vi "Wait for Record Event.vi"(6 "Cancel":bool, 8 "error in":errorcluster, 9 "Timeout in ms (0: infinite)":u32, 10 "Event":u16(ring)=32 items=["Record Start"=32, "Record End"=64, "Start Trigger"=128], 11 "VISA resource name":refnum<visa-resource-name>) -> (0 "error out":errorcluster, 3 "VISA resource name out":refnum<visa-resource-name>)   [LabVIEW 2017, in "Sefram DAS220.lvlib"]
doc: "Wait for record event : start, end or start trigger."
uses:
  <instrlib>/Sefram DAS220/Sefram DAS220.lvlib
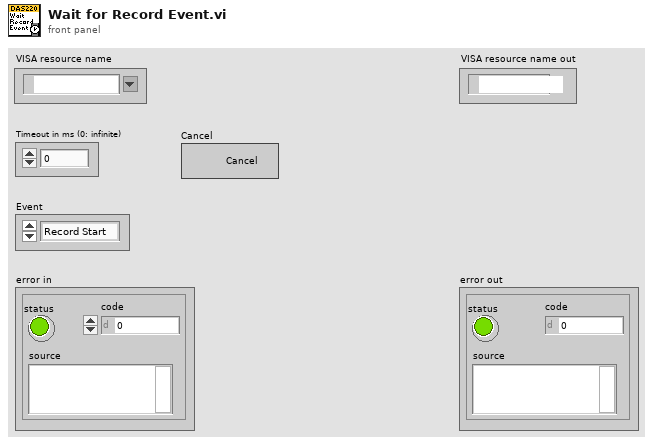
[diagram p1: front panel]
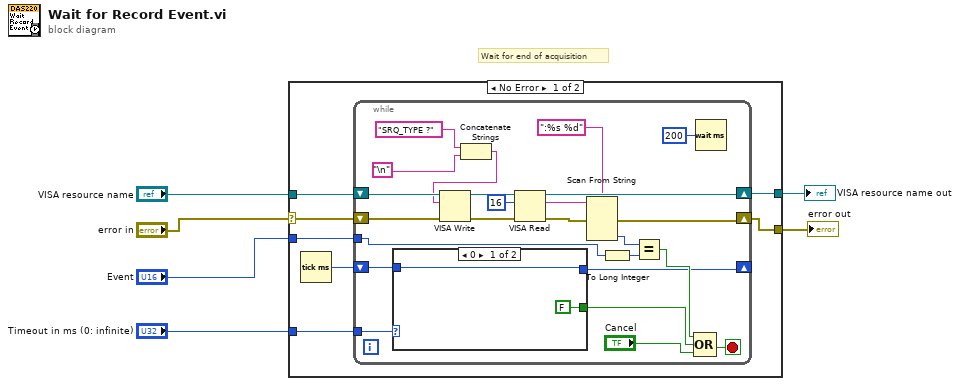
[diagram p0: block diagram]
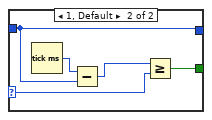
[diagram p2: hidden frame]
diagram:
  # "Wait for end of acquisition"
  n1 = case shown="No Error" "error in" {
    selector: "error in" -> [w7 w45]
    tunnel: "Timeout in ms (0: infinite)" -> [w12 _]
    tunnel: "VISA resource name" -> [w11 w46]
    tunnel: [w10 w46] -> w4
    tunnel: [w9 w45] -> w3
    tunnel: "Event" -> [w8 _]
    frame No Error {
      n2 = Tick Count (ms)() -> (millisecond timer value=w13:u32)
      n3 = while {
        shift-right: [w31] -> w10
        shift-left: w11 -> [w36]
        shift-right: [w24] -> w9
        shift-left: w7 -> [w35]
        shift-right: [w17] -> _
        shift-left: w13 -> [w18]
        tunnel: w12 -> [w19]
        tunnel: w8 -> [w15]
        stop <- w20 stop-if-true
        n4 = case shown="0" w19 {
          selector: w19 -> [_ w41]
          tunnel: w18 -> [w39 w43]
          tunnel: [w39 w43] -> w17
          tunnel: [FALSE w40] -> w16
          frame 0 {
          }
          frame 1, Default {
            n5 = Tick Count (ms)() -> (millisecond timer value=w44:u32)
            n6 = Subtract(x=w44, y=w43) -> (x-y=w42:u32)
            n7 = Greater Or Equal?(x=w42, y=w41) -> (x >= y?=w40:bool)
          }
        }
        n8 = Concatenate Strings("SRQ_TYPE ?" ("write buffer"), "\n") -> (w33:string)
        n9 = VISA Write(VISA resource name=w36, write buffer=w33, error in (no error)=w35) -> (VISA resource name out=w32:refnum<visa-resource-name>, error out=w30:errorcluster)  [unwired: 1 out]
        n10 = VISA Read(VISA resource name=w32, byte count=u32 16, error in (no error)=w30) -> (VISA resource name out=w31:refnum<visa-resource-name>, read buffer=w26:string, error out=w25:errorcluster)  [unwired: 1 out]
        n11 = Scan From String(format string=":%s %d", input string=w26, error in=w25) -> (error out=w24:errorcluster, output 2=w23:i32)  [unwired: 4 in, 2 out]
        n12 = To Long Integer(number=w15) -> (32bit integer=w14:i32)
        n13 = Equal?(x=w23, y=w14) -> (x = y?=w22:bool)
        n14 = Compound Arithmetic op=OR(w22, w16, "Cancel") -> (w20:bool)
        n15 = Wait (ms)(milliseconds to wait=u32 200) -> ()  [unwired: 1 out]
      }
    }
    frame Error {
    }
  }
  "VISA resource name out" <- w4
  "error out" <- w3
